vi "Transform.vi"(8 "error in (no error)":errorcluster caption="entrée d'erreur (pas d'erreur)", 9 "y":string[][](array[string]), 10 "X":string[][](array[string]), 11 "KBinsDiscretizer.lvclass":refnum<class "KBinsDiscretizer.lvclass">) -> (0 "error out":errorcluster caption="sortie d'erreur", 2 "Data":T1, 3 "KBinsDiscretizer.lvclass":refnum<class "KBinsDiscretizer.lvclass">)   [LabVIEW 2020, in "KBinsDiscretizer.lvclass"]
doc: "Discretize the data.\n\nReturns : \n\n- Xt : numeric array-like or sparse matrix\nData in the binned space."
uses:
  KBinsDiscretizer.lvclass
  KBinsDiscretizer.lvclass/KBinsDiscretizer.ctl
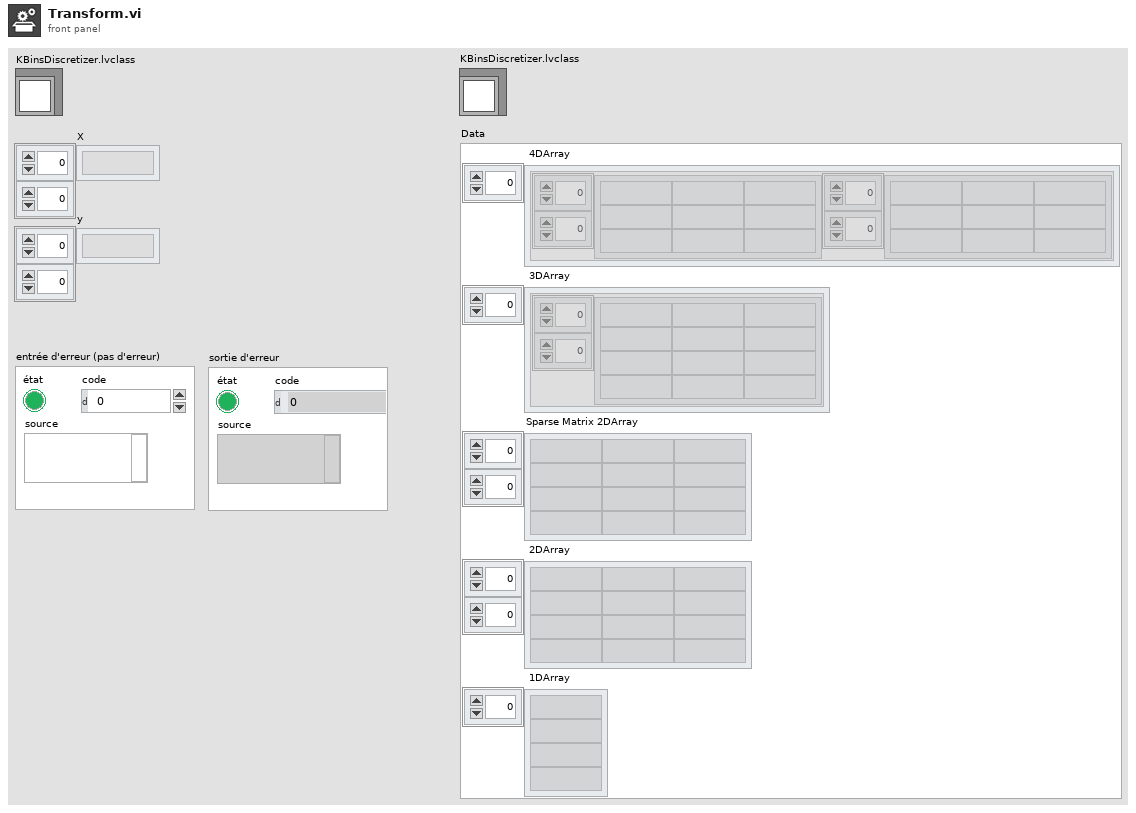
[diagram p1: front panel]
types:
  T1 = cluster{" 4DArray":cluster{"1":string[][], "2":string[][]}[], " 3DArray":cluster{"Tableau":string[][]}[], "Sparse Matrix 2DArray":string[][], " 2DArray":string[][], " 1DArray":string[]}
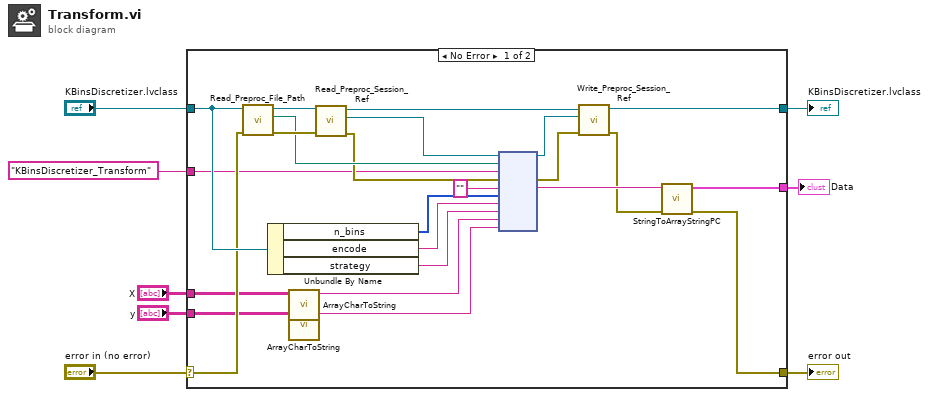
[diagram p0: block diagram]
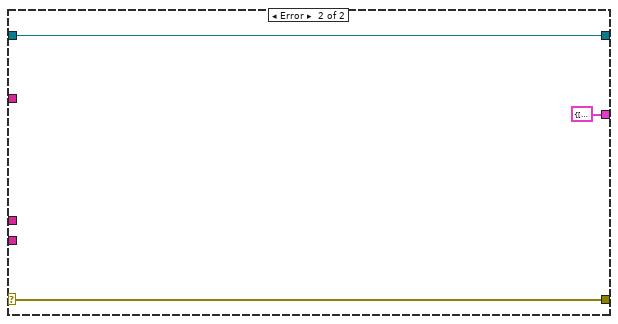
[diagram p2: hidden frame]
diagram:
  n1 = case shown="No Error" "error in (no error)" {
    selector: "error in (no error)" -> [w22 w35]
    tunnel: [w10 w35] -> w7
    tunnel: [w12 w34] -> w5
    tunnel: "KBinsDiscretizer.lvclass" -> [w23 w34]
    tunnel: "KBinsDiscretizer_Transform" ("Fonction") -> [w18 _]
    tunnel: [w9 T1 {" 4DArray"=[], " 3DArray"=[], "Sparse Matrix 2DArray"=[], " 2DArray"=[], " 1DArray"=[]} ("Data")] -> w1
    tunnel: "X" -> [w17 _]
    tunnel: "y" -> [w16 _]
    frame No Error {
      n2 = call-dynamic "Read_Preproc_File_Path.vi"("error in (no error)"=w22, "Python in"=w23) -> ("error out"=w31:errorcluster, "File_Path"=w28:path, "Python out"=w32:refnum<class "KBinsDiscretizer.lvclass">)  [unwired: 7 in]
      n3 = Unbundle By Name(w23) -> ("n_bins"=w21:i32[], "encode"=w20:string, "strategy"=w19:string)
      n4 = call "ArrayCharToString.vi"("TAB"=w17) -> ("Instruction"=w15:string)  [unwired: 10 in]
      n5 = call "ArrayCharToString.vi"("TAB"=w16) -> ("Instruction"=w14:string)  [unwired: 10 in]
      n6 = call-dynamic "Read_Preproc_Session_Ref.vi"("error in (no error)"=w31, "Python in"=w32) -> ("error out"=w27:errorcluster, "Session_ref"=w29:refnum<k35>, "Python out"=w30:refnum<class "KBinsDiscretizer.lvclass">)  [unwired: 7 in]
      n7 = node(w29, w28, w18, w27, "", w21, w20, w19, w15, w14) -> (w25:refnum<k35>, w26:errorcluster, w13:string)  [unwired: 5 in, 2 out]
      n8 = call-dynamic "Write_Preproc_Session_Ref.vi"("error in (no error)"=w26, "Session_ref"=w25, "Python in"=w30) -> ("error out"=w11:errorcluster, "Python out"=w12:refnum<class "KBinsDiscretizer.lvclass">)  [unwired: 7 in]
      n9 = call "StringToArrayStringPC.vi"("sortie d'erreur"=w11, "Return value"=w13) -> ("sortie d'erreur"=w10:errorcluster, "Data"=w9:T1)  [unwired: 8 in]
    }
    frame Error {
    }
  }
  "error out" <- w7
  "KBinsDiscretizer.lvclass" <- w5
  "Data" <- w1
